vi "sm bool write and increment.vi"(9 "Identifier":string, 10 "value in":bool, 11 "Shared memory cluster input":T1) -> (3 "Shared memory cluster output":T1)   [LabVIEW 2018, in "linuxSharedMemory.lvlib"]
uses:
  linuxSharedMemory.lvlib
  controls/sm_cluster.ctl
  <vilib>/NI/NI Linux RT IPC/Shared Memory/Pointer Operations/Write Scalar Boolean.vi
  <vilib>/NI/NI Linux RT IPC/Shared Memory/Linux RT IPC.Shared Memory.lvlib
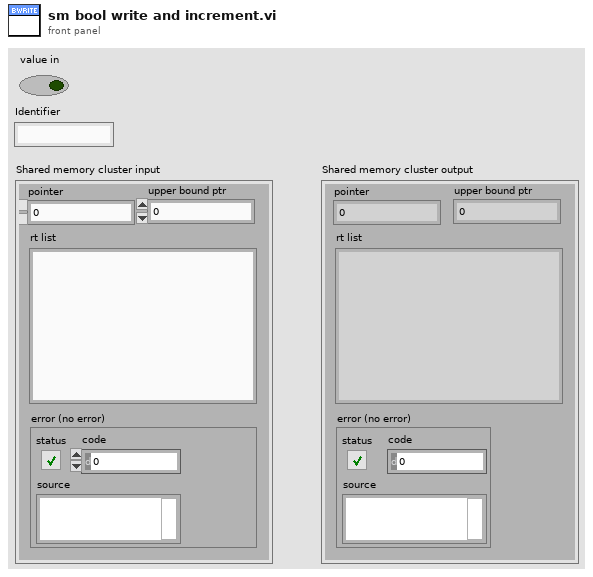
[diagram p1: front panel]
types:
  T1 = typedef "linuxSharedMemory.lvlib/sm_cluster.ctl" = cluster{"rt list":string, "error (no error)":errorcluster, "pointer":u64, "upper bound ptr":u64}
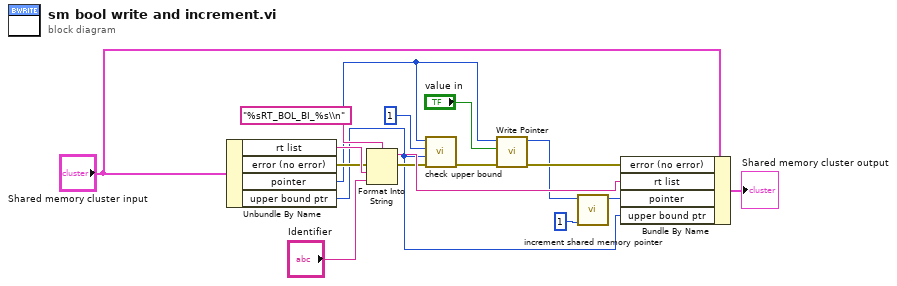
[diagram p0: block diagram]
diagram:
  n1 = Unbundle By Name("Shared memory cluster input") -> ("rt list"=w12:string, "error (no error)"=w9:errorcluster, "pointer"=w2:u64, "upper bound ptr"=w6:u64)
  n2 = Format Into String(format string="%sRT_BOL_BI_%s\\n", error in=w9, w12, "Identifier") -> (resulting string=w10:string, error out=w8:errorcluster)  [unwired: 1 in]
  n3 = call "check upper bound.vi"("error in (no error)"=w8, "ptr upper bound (inclusive)"=w6, "size"=1, "ptr in"=w2) -> ("error out"=w4:errorcluster)  [unwired: 7 in]
  n4 = call-poly <vilib>:"Write Pointer.vi"("error in (no error)"=w4, "value"="value in", "pointer in"=w2) -> ("error out"=w3:errorcluster, "pointer out"=w1:u64)  [unwired: 6 in, 1 out]
  n5 = call "increment shared memory pointer.vi"("Increment value"=1, "Shared Memory PTR in"=w1) -> ("Shared Memory PTR out"=w7:u64)  [unwired: 9 in]
  n6 = Bundle By Name(cluster="Shared memory cluster input", "error (no error)"=w3, "rt list"=w10, "pointer"=w7, "upper bound ptr"=w6) -> (→"Shared memory cluster output":T1)
